vi "Stop Acquisition.vi"(8 "error in":errorcluster, 11 "5105 in":refnum<class "5105.lvclass">) -> (0 "error out":errorcluster, 3 "5105 out":refnum<class "5105.lvclass">)   [LabVIEW 2019, in "5105.lvlib" / "5105.lvclass"]
uses:
  5105.lvclass
  Accessors/Read Local Resource.vi
  Accessors/Write Local Resource.vi
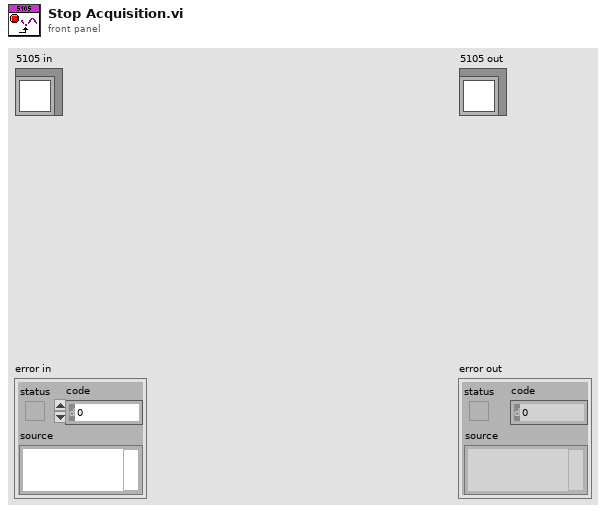
[diagram p1: front panel]
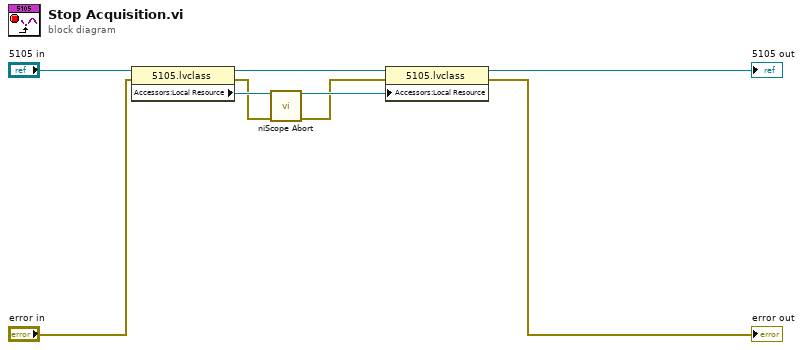
[diagram p0: block diagram]
diagram:
  n1 = property class="5105.lvclass"(reference="5105 in", error in="error in") -> (reference out=w7:refnum<class "5105.lvclass">, error out=w5:errorcluster, "Accessors:Local Resource"=w8:refnum<k15>)
  n2 = call <instrlib>:"niScope Abort.vi"("instrument handle"=w8, "error in"=w5) -> ("instrument handle out"=w6:refnum<k15>, "error out"=w4:errorcluster)  [unwired: 12 in]
  n3 = property class="5105.lvclass"(reference=w7, error in=w4, "Accessors:Local Resource"=w6) -> (reference out=→"5105 out":refnum<class "5105.lvclass">, error out=→"error out":errorcluster)
